vi "Data.vi"(7 "LWRS":refnum<class "Web Request.lvclass">) -> ()   [LabVIEW 2014]
uses:
  <vilib>/wsapi/Web Request.lvclass
  Controller/Controls/Notifier Enum.ctl
  reusable/Data/Data.lvclass
  reusable/Data/Read measTime.vi
  Controller/Controller.lvclass
panel:
  out "Array":errorcluster[](array[cluster])
  out "String":string
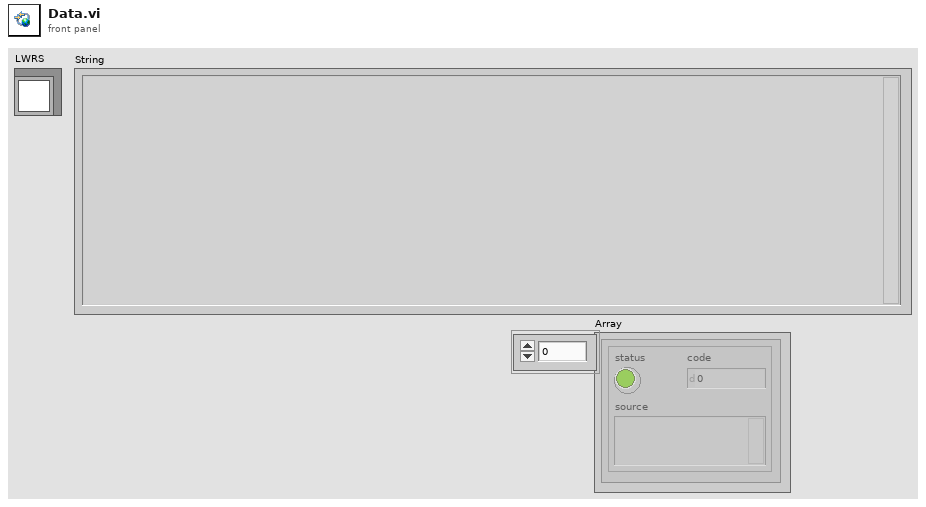
[diagram p1: front panel]
types:
  T1 = typedef "Controller.lvlib/Controller.lvclass/Notifier Enum.ctl" = enum16{"Initialize", "Get", "Set", "Close"}
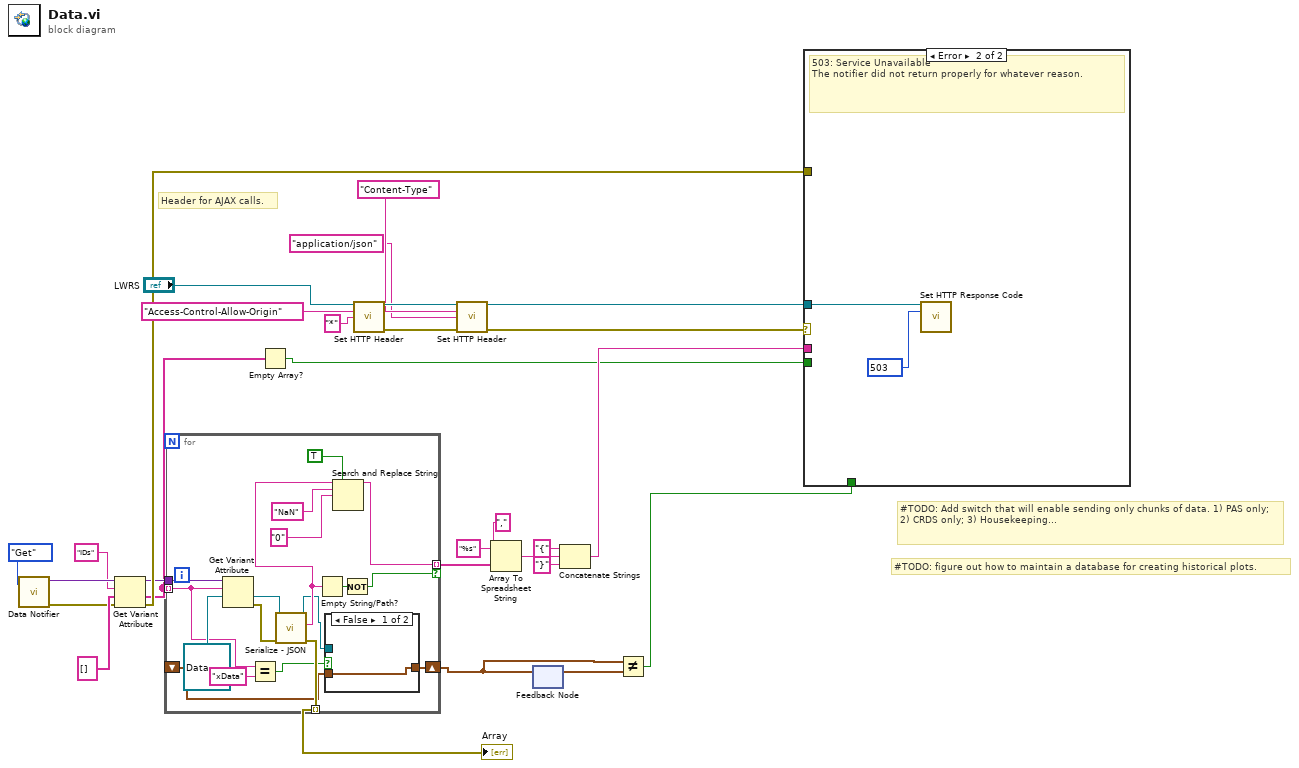
[diagram p0: block diagram]
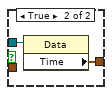
[diagram p2: hidden frame]
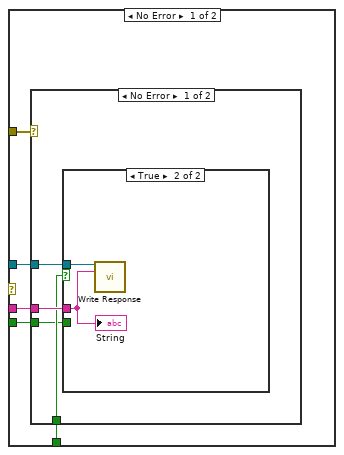
[diagram p3: hidden frame]
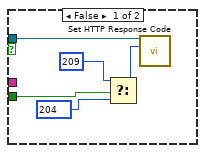
[diagram p4: hidden frame]
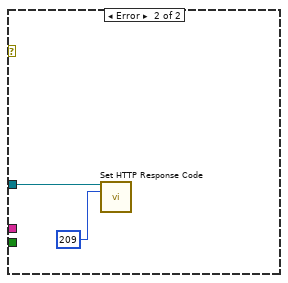
[diagram p5: hidden frame]
diagram:
  # "#TODO: figure out how to maintain a database for creating historical plots."
  # "#TODO: Add switch that will enable sending only chunks of data. 1) PAS only; 2) CRDS only; 3) Housekeeping..."
  # "Header for AJAX calls."
  n1 = call "Data Notifier.vi"("State"=Notifier_Enum."Get") -> ("error out"=w8:errorcluster, "Data Map"=w18:variant)  [unwired: 9 in]
  n2 = Get Variant Attribute(Variant=w18, name="IDs", default value (empty Variant)=string[] [], error in=w8) -> (duplicate Variant=w15:variant, value=w5:string[], error out=w20:errorcluster)  [unwired: 1 out]
  n3 = for {
    tunnel: w5 -> [w35] mode=indexing
    tunnel: w15 -> [w47]
    tunnel: [w36] -> w14 mode=indexing if=w43
    tunnel: [w41] -> w7 mode=indexing
    shift-right: [w31] -> w3
    shift-left: _ -> [w30]
    n4 = Get Variant Attribute(Variant=w47, name=w35, default value (empty Variant)=refnum<class "Data.lvclass"> refnum ("Base Data Lib:Data")) -> (value=w45:refnum<class "Data.lvclass">, error out=w42:errorcluster)  [unwired: 1 in, 2 out]
    n5 = Equal?(x=w35, y="xData") -> (x = y?=w33:bool)
    n6 = call-dynamic "Serialize - JSON.vi"("error in"=w42, "Data in"=w45) -> ("error out"=w41:errorcluster, "Serialized JSON"=w37:string, "Data out"=w32:refnum<class "Data.lvclass">)  [unwired: 7 in]
    n7 = Empty String/Path?(string/path=w37) -> (empty?=w44:bool)
    n8 = case shown="False" w33 {
      tunnel: w32 -> [_ w50]
      tunnel: [w48 w49] -> w31
      tunnel: w30 -> [w48 _]
      frame False {
      }
      frame True {
        n9 = property class="Data"(reference=w50) -> ("Time"=w49:timestamp)  [unwired: 1 in, 2 out]
      }
    }
    n10 = Search and Replace String(replace all?=TRUE ("replace all? (F)"), input string=w37, search string="NaN", replace string="0" ("replace string (\"\")")) -> (result string=w36:string)  [unwired: 4 in, 3 out]
    n11 = Not(x=w44) -> (.not. x?=w43:bool)
  }
  "Array" <- w7
  n12 = Empty Array?(array=w5) -> (empty?=w4:bool)
  n13 = call <vilib>:"Set HTTP Header.vi"("LabVIEW Web Service Request"="LWRS", "header"="Access-Control-Allow-Origin", "header value"="*") -> ("LabVIEW Web Service Request out"=w27:refnum<class "Web Request.lvclass">, "error out"=w26:errorcluster)  [unwired: 11 in]
  n14 = call <vilib>:"Set HTTP Header.vi"("LabVIEW Web Service Request"=w27, "header"="Content-Type", "header value"="application/json", "error in (no error)"=w26) -> ("LabVIEW Web Service Request out"=w22:refnum<class "Web Request.lvclass">, "error out"=w25:errorcluster)  [unwired: 10 in]
  n15 = Array To Spreadsheet String(delimiter (Tab)=",", array=w14, 3:"%s" ("format string")) -> (spreadsheet string=w11:string)
  n16 = feedback-in #1(w3) -> ()
  n17 = feedback #1() -> (w2:timestamp)  [unwired: 1 in]
  n18 = Concatenate Strings("{" ("string"), w11, "}" ("string")) -> (w6:string)
  n19 = Not Equal?(x=w3, y=w2) -> (x != y?=w1:bool)
  n20 = case shown="Error" w25 {
    tunnel: w20 -> [w55 _]
    tunnel: w22 -> [w54 w70]
    tunnel: w6 -> [w53 _]
    tunnel: w1 -> [w52 _]
    tunnel: w4 -> [w51 _]
    frame No Error {
      n21 = case shown="No Error" w55 {
        tunnel: w54 -> [w59 w68]
        tunnel: w53 -> [w58 _]
        tunnel: w52 -> [w57 _]
        tunnel: w51 -> [w56 _]
        frame No Error {
          # "200: OK"
          n22 = case shown="True" w57 {
            tunnel: w59 -> [w64 w66]
            tunnel: w58 -> [_ w65]
            tunnel: w56 -> [w63 _]
            frame False {
              w62 = 204 items=["100"=100, "101"=101, "200"=200, "201"=201, "202"=202, "203"=203, "204"=204, "205"=205, "206"=206, "300"=300, "301"=301, "302"=302, "303"=303, "304"=304, "305"=305, "306"=306, "307"=307, "400"=400, "401"=401, "402"=402, "403"=403, "404"=404, "405"=405, "406"=406, "407"=407, "408"=408, "409"=409, "410"=410, "411"=411, "412"=412, "413"=413, "414"=414, "415"=415, "416"=416, "417"=417, "500"=500, "501"=501, "502"=502, "503"=503, "504"=504, "505"=505] ("response code (200)")
              n23 = Select(t=209, s=w63, f=w62) -> (s? t:f=w60:i32)
              n24 = call <vilib>:"Set HTTP Response Code.vi"("LabVIEW Web Service Request"=w64, "response code (200)"=w60) -> ()  [unwired: 12 in, 2 out]
            }
            frame True {
              n25 = call <vilib>:"Write Response.vi"("LabVIEW Web Service Request"=w66, "response string"=w65) -> ()  [unwired: 12 in, 2 out]
              "String" <- w65
            }
          }
        }
        frame Error {
          # "204: No Content\nService is valid, DVR is broken"
          n26 = call <vilib>:"Set HTTP Response Code.vi"("LabVIEW Web Service Request"=w68, "response code (200)"=209) -> ()  [unwired: 12 in, 2 out]
        }
      }
    }
    frame Error {
      w69 = 503 items=["100"=100, "101"=101, "200"=200, "201"=201, "202"=202, "203"=203, "204"=204, "205"=205, "206"=206, "300"=300, "301"=301, "302"=302, "303"=303, "304"=304, "305"=305, "306"=306, "307"=307, "400"=400, "401"=401, "402"=402, "403"=403, "404"=404, "405"=405, "406"=406, "407"=407, "408"=408, "409"=409, "410"=410, "411"=411, "412"=412, "413"=413, "414"=414, "415"=415, "416"=416, "417"=417, "500"=500, "501"=501, "502"=502, "503"=503, "504"=504, "505"=505] ("response code (200)")
      # "503: Service Unavailable\nThe notifier did not return properly for whatever reason."
      n27 = call <vilib>:"Set HTTP Response Code.vi"("LabVIEW Web Service Request"=w70, "response code (200)"=w69) -> ()  [unwired: 12 in, 2 out]
    }
  }
